vi "Q5 Format.vi"(11 "Data (U16 or U32)":string) -> (3 "Q5 Format Data":string)   [LabVIEW 2016, in "GEA2_Toolkit.lvlib"]
uses:
  library/GEA2_Toolkit.lvlib
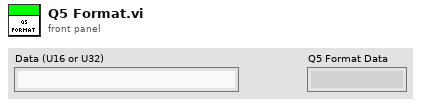
[diagram p1: front panel]
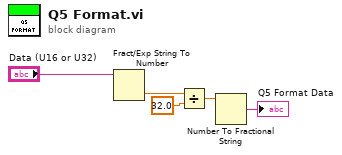
[diagram p0: block diagram]
diagram:
  n1 = Fract/Exp String To Number(string="Data (U16 or U32)") -> (number=w5:dbl)  [unwired: 3 in, 1 out]
  n2 = Divide(x=w5, y=32.0) -> (x/y=w2:dbl)
  n3 = Number To Fractional String(number=w2) -> (F-format string=→"Q5 Format Data":string)  [unwired: 3 in]
